vi "ActDriveStraightFast.vi"(9 "FirstTime":bool, 10 "MaxSpeed (ft/s)":dbl, 11 "Dist (ft)":dbl) -> (0 "RightSpeedDemand":dbl, 1 "LeftSpeedDemand":dbl, 3 "Done":bool)   [LabVIEW 2020]
doc: "Robot will drive forward straight a set distance utilizing position control \n\nInputs:\n-- MaxSpeed -- Double -- in ft/s, the MaxSpeed the robot can go -- \n-- Dist (ft) -- Double -- Distance in feet you want the robot to go -- \n-- FirstTime -- Boolean -- Input true the first time this function is called, sets the target position -- \n\nOutputs:\n-- Done -- Bool -- has the robot reached its target distance\n-- LeftSpeedDemand -- Double -- Speed Demand for left drive train inorder to reach target -- \n-- RightSpeedDemand -- Double -- Speed Demand for left drive train inorder to reach target --"
uses:
  <vilib>/Rock Robotics/Network Tables/NT Write Boolean.vi
  <vilib>/Rock Robotics/Network Tables/NT Write Number.vi
  <vilib>/Rock Robotics/WPI/ThirdParty/JAS_Junk/TrajLib/Trajectory_Library.lvlib
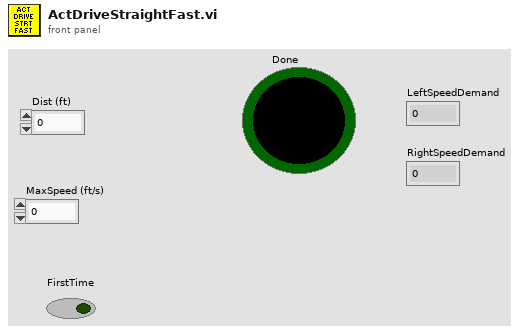
[diagram p1: front panel]
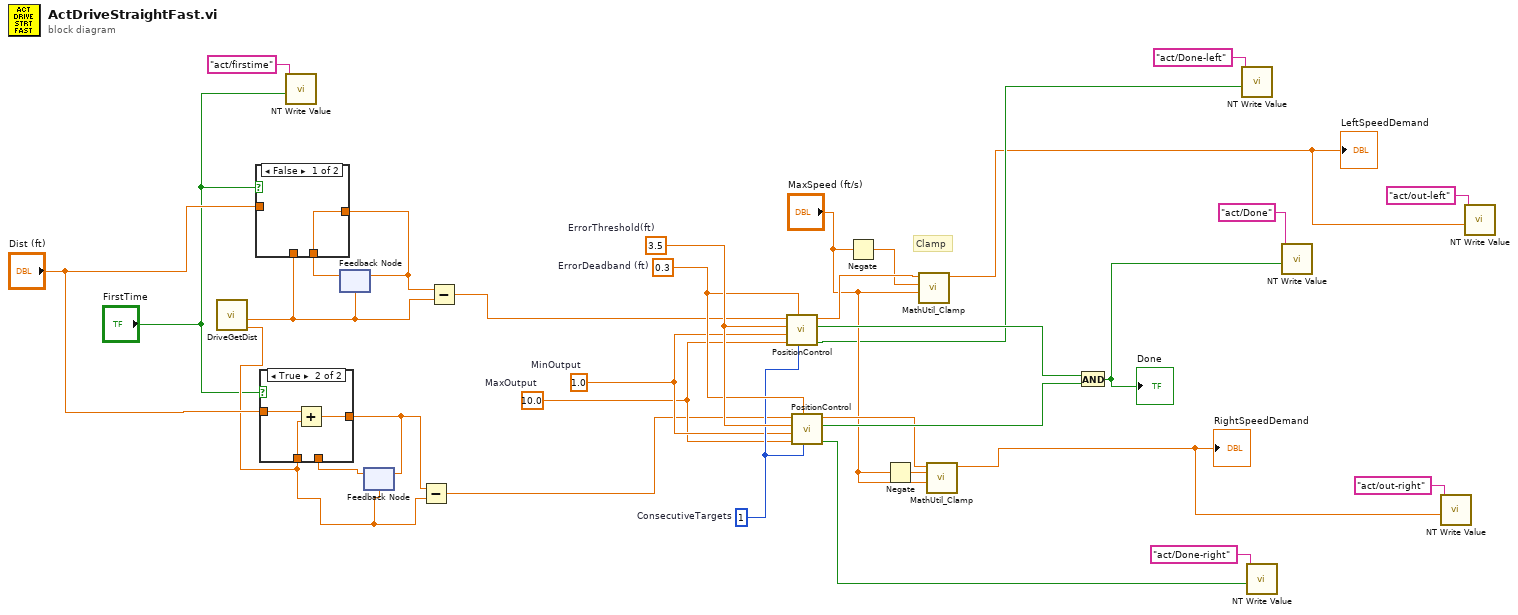
[diagram p0: block diagram]
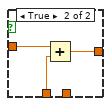
[diagram p3: hidden frame]
diagram:
  w14 = 10.0  # MaxOutput
  w15 = 1.0  # MinOutput
  w26 = 1  # ConsecutiveTargets
  w29 = 0.3  # ErrorDeadband (ft)
  w30 = 3.5  # ErrorThreshold(ft)
  # "Clamp"
  n1 = call "DriveGetDist.vi"() -> ("Right dist"=w20:dbl, "Left dist"=w18:dbl)  [unwired: 10 in]
  n2 = call-poly <vilib>:"NT Write Value.vi"("value"="FirstTime", "name"="act/firstime") -> ()  [unwired: 9 in, 1 out]
  n3 = feedback #1(w18) -> (w32:dbl)
  n4 = case shown="False" "FirstTime" {
    tunnel: "Dist (ft)" -> [_ w37]
    tunnel: w18 -> [_ w36]
    tunnel: [w34 w35] -> w19
    tunnel: w32 -> [w34 _]
    frame False {
    }
    frame True {
      n5 = Add(x=w37, y=w36) -> (x+y=w35:dbl)
    }
  }
  n6 = feedback-in #1(w19) -> ()
  n7 = feedback #2(w20) -> (w31:dbl)
  n8 = case shown="True" "FirstTime" {
    tunnel: "Dist (ft)" -> [_ w41]
    tunnel: w20 -> [_ w40]
    tunnel: [w38 w39] -> w11
    tunnel: w31 -> [w38 _]
    frame False {
    }
    frame True {
      n9 = Add(x=w41, y=w40) -> (x+y=w39:dbl)
    }
  }
  n10 = feedback-in #2(w11) -> ()
  n11 = Subtract(x=w11, y=w20) -> (x-y=w13:dbl)
  n12 = Subtract(x=w19, y=w18) -> (x-y=w12:dbl)
  n13 = call "PositionControl.vi"("ConsecutiveTargets"=w26, "ErrorDeadband"=w29, "MaxOutput"=w14, "MinOutput"=w15, "ErrorThreshold"=w30, "Error"=w12) -> ("UnfilteredOnTarget"=w7:bool, "OnTarget"=w27:bool, "OutputValue"=w25:dbl)  [unwired: 3 in]
  n14 = call "PositionControl.vi"("ConsecutiveTargets"=w26, "ErrorDeadband"=w29, "MaxOutput"=w14, "MinOutput"=w15, "ErrorThreshold"=w30, "Error"=w13) -> ("UnfilteredOnTarget"=w8:bool, "OnTarget"=w28:bool, "OutputValue"=w23:dbl)  [unwired: 3 in]
  n15 = Negate(x="MaxSpeed (ft/s)") -> (-x=w24:dbl)
  n16 = Negate(x="MaxSpeed (ft/s)") -> (-x=w22:dbl)
  n17 = call <vilib>:"MathUtil_Clamp.vi"("High Limit"="MaxSpeed (ft/s)", "Low Limit"=w24, "Value"=w25) -> ("Result"=w5:dbl)  [unwired: 8 in]
  "LeftSpeedDemand" <- w5
  n18 = call <vilib>:"MathUtil_Clamp.vi"("High Limit"="MaxSpeed (ft/s)", "Low Limit"=w22, "Value"=w23) -> ("Result"=w3:dbl)  [unwired: 8 in]
  "RightSpeedDemand" <- w3
  n19 = And(x=w27, y=w28) -> (x .and. y?=w16:bool)
  "Done" <- w16
  n20 = call-poly <vilib>:"NT Write Value.vi"("value"=w7, "name"="act/Done-left") -> ()  [unwired: 9 in, 1 out]
  n21 = call-poly <vilib>:"NT Write Value.vi"("value"=w8, "name"="act/Done-right") -> ()  [unwired: 9 in, 1 out]
  n22 = call-poly <vilib>:"NT Write Value.vi"("value"=w16, "name"="act/Done") -> ()  [unwired: 9 in, 1 out]
  n23 = call-poly <vilib>:"NT Write Value.vi"("value"=w3, "name"="act/out-right") -> ()  [unwired: 9 in, 1 out]
  n24 = call-poly <vilib>:"NT Write Value.vi"("value"=w5, "name"="act/out-left") -> ()  [unwired: 9 in, 1 out]
